vi "UpdateUserInterface.vi"(8 "error in (no error)":errorcluster, 10 "DataExchange":T2, 11 "MicroscopeController in":refnum<class "MicroscopeController.lvclass">) -> (0 "error out":errorcluster, 2 "DataExchange Out":T2, 3 "MicroscopeController out":refnum<class "MicroscopeController.lvclass">)   [LabVIEW 2020, in "MicroscopeController.lvlib" / "MicroscopeController.lvclass"]
uses:
  MicroscopeController.lvclass
  Model/Hardware Abstraction Layer/Component/Device/Device/DataExchange.ctl
  MicroscopeController.lvclass/MicroscopeController.ctl
  Model/Hardware Abstraction Layer/Component/GenericActor/GenericActor/GenericController.lvclass
  Interface/DataListener/DataListener.lvclass
panel:
  in  "cluster":T1
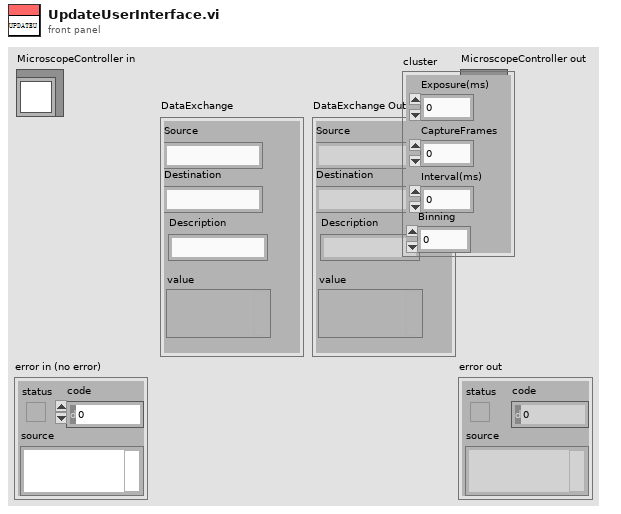
[diagram p1: front panel]
types:
  T1 = cluster{"Exposure(ms)":dbl, "CaptureFrames":dbl, "Interval(ms)":dbl, "Binning":dbl}
  T2 = typedef "DataListener.lvclass/DataExchange.ctl" = cluster{"Source":string, "Destination":string, "Description":string, "value":variant}
  T3 = enum32{"Invalid", "Standard", "Closed", "Hidden", "Minimized", "Maximized"}
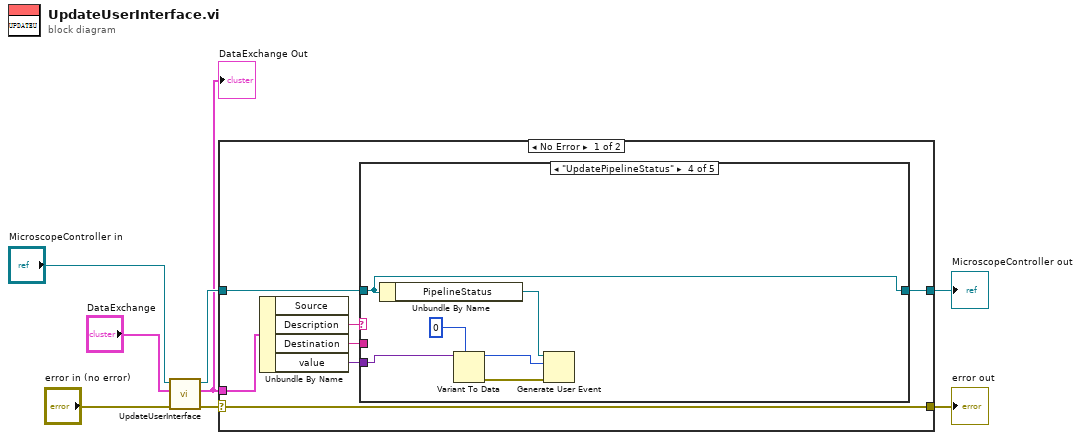
[diagram p0: block diagram]
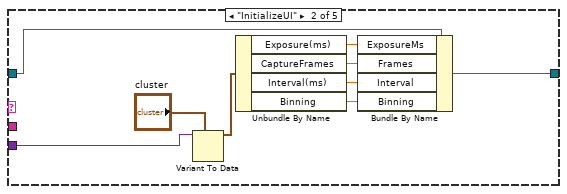
[diagram p3: hidden frame]
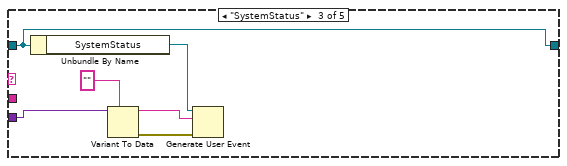
[diagram p4: hidden frame]
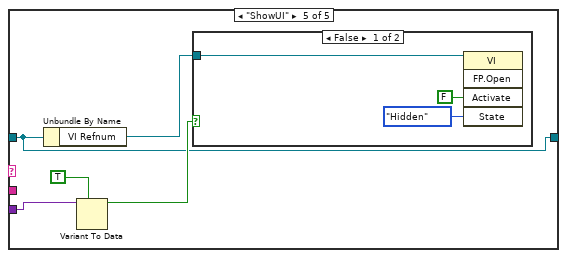
[diagram p5: hidden frame]
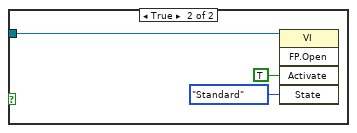
[diagram p6: hidden frame]
diagram:
  n1 = call-parent "UpdateUserInterface.vi"("error in (no error)"="error in (no error)", "DataExchange"="DataExchange", "GenericController in"="MicroscopeController in") -> ("error out"=w4:errorcluster, "DataExchange Out"=w1:T2, "GenericController out"=w5:refnum<class "MicroscopeController.lvclass">)  [unwired: 6 in]
  "DataExchange Out" <- w1
  n2 = case shown="No Error" w4 {
    selector: w4 -> [w15 w50]
    tunnel: [w15 w50] -> w2
    tunnel: [w9 w49] -> w3
    tunnel: w5 -> [w10 w49]
    tunnel: w1 -> [w14 _]
    frame No Error {
      n3 = Unbundle By Name(w14) -> ("Description"=w11:string, "Destination"=w12:string, "value"=w13:variant)  [unwired: 1 out]
      n4 = case shown="\"UpdatePipelineStatus\"" w11 {
        tunnel: w13 -> [_ w24 w31 w37 w42]
        tunnel: w12 -> [_ _ _ _ _]
        tunnel: w10 -> [w16 w25 w26 w34 w38]
        tunnel: [w16 w23 w26 w34 w38] -> w9
        frame Default {
        }
        frame "InitializeUI" {
          n5 = Variant To Data(type="cluster", Variant=w24) -> (data=w22:T1)  [unwired: 1 in, 1 out]
          n6 = Unbundle By Name(w22) -> ("Exposure(ms)"=w21:dbl, "CaptureFrames"=w20:dbl, "Interval(ms)"=w19:dbl, "Binning"=w17:dbl)
          n7 = Bundle By Name(cluster=w25, "ExposureMs"=w21, "Frames"=w20, "Interval"=w19, "Binning"=w17) -> (w23:refnum<class "MicroscopeController.lvclass">)
        }
        frame "SystemStatus" {
          n8 = Unbundle By Name(w26) -> ("SystemStatus"=w30:refnum<user-event>)
          n9 = Variant To Data(type="" ("event data"), Variant=w31) -> (data=w27:string, error out=w29:errorcluster)  [unwired: 1 in]
          n10 = Generate User Event(user event=w30, event data cluster=w27, error in=w29) -> ()  [unwired: 1 in, 2 out]
        }
        frame "UpdatePipelineStatus" {
          n11 = Unbundle By Name(w34) -> ("PipelineStatus"=w36:refnum<user-event>)
          n12 = Variant To Data(type=u8 0 ("event data"), Variant=w37) -> (data=w32:u8, error out=w35:errorcluster)  [unwired: 1 in]
          n13 = Generate User Event(user event=w36, event data cluster=w32, error in=w35) -> ()  [unwired: 1 in, 2 out]
        }
        frame "ShowUI" {
          n14 = Unbundle By Name(w38) -> ("VI Refnum"=w39:refnum<vi>)
          n15 = Variant To Data(type=TRUE, Variant=w42) -> (data=w40:bool)  [unwired: 1 in, 1 out]
          n16 = case shown="False" w40 {
            tunnel: w39 -> [w45 w48]
            frame False {
              n17 = invoke class="VI" method="FP.Open"(reference=w45, "Activate"=FALSE ("Activate?"), "State"=T3."Hidden") -> ()  [unwired: 2 in, 5 out]
            }
            frame True {
              n18 = invoke class="VI" method="FP.Open"(reference=w48, "Activate"=TRUE ("Activate?"), "State"=T3."Standard") -> ()  [unwired: 2 in, 5 out]
            }
          }
        }
      }
    }
    frame Error {
    }
  }
  "error out" <- w2
  "MicroscopeController out" <- w3
